vi "ViGmentize.vi"() -> ()   [LabVIEW 2025]
panel:
  in  "Style":T1(ring)=enum."material"
  in  "ACTION":bool
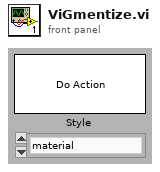
[diagram p1: front panel]
types:
  T1 = enum16{"abap", "algol", "algol_nu", "arduino", "autumn", "bw", "borland", "coffee", "colorful", "default", "dracula", "emacs", "friendly_grayscale", "friendly", "fruity", "github-dark", "gruvbox-dark", "gruvbox-light", "igor", "inkpot", "lightbulb", "lilypond", "lovelace", "manni", "material", "monokai", "murphy", "native", "nord-darker", "nord", "one-dark", "paraiso-dark", "paraiso-light", "pastie", "perldoc", "rainbow_dash", "rrt", "sas", "solarized-dark", "solarized-light", "staroffice", "stata-dark", "stata-light", "tango", "trac", "vim", "vs", "xcode", "zenburn"}
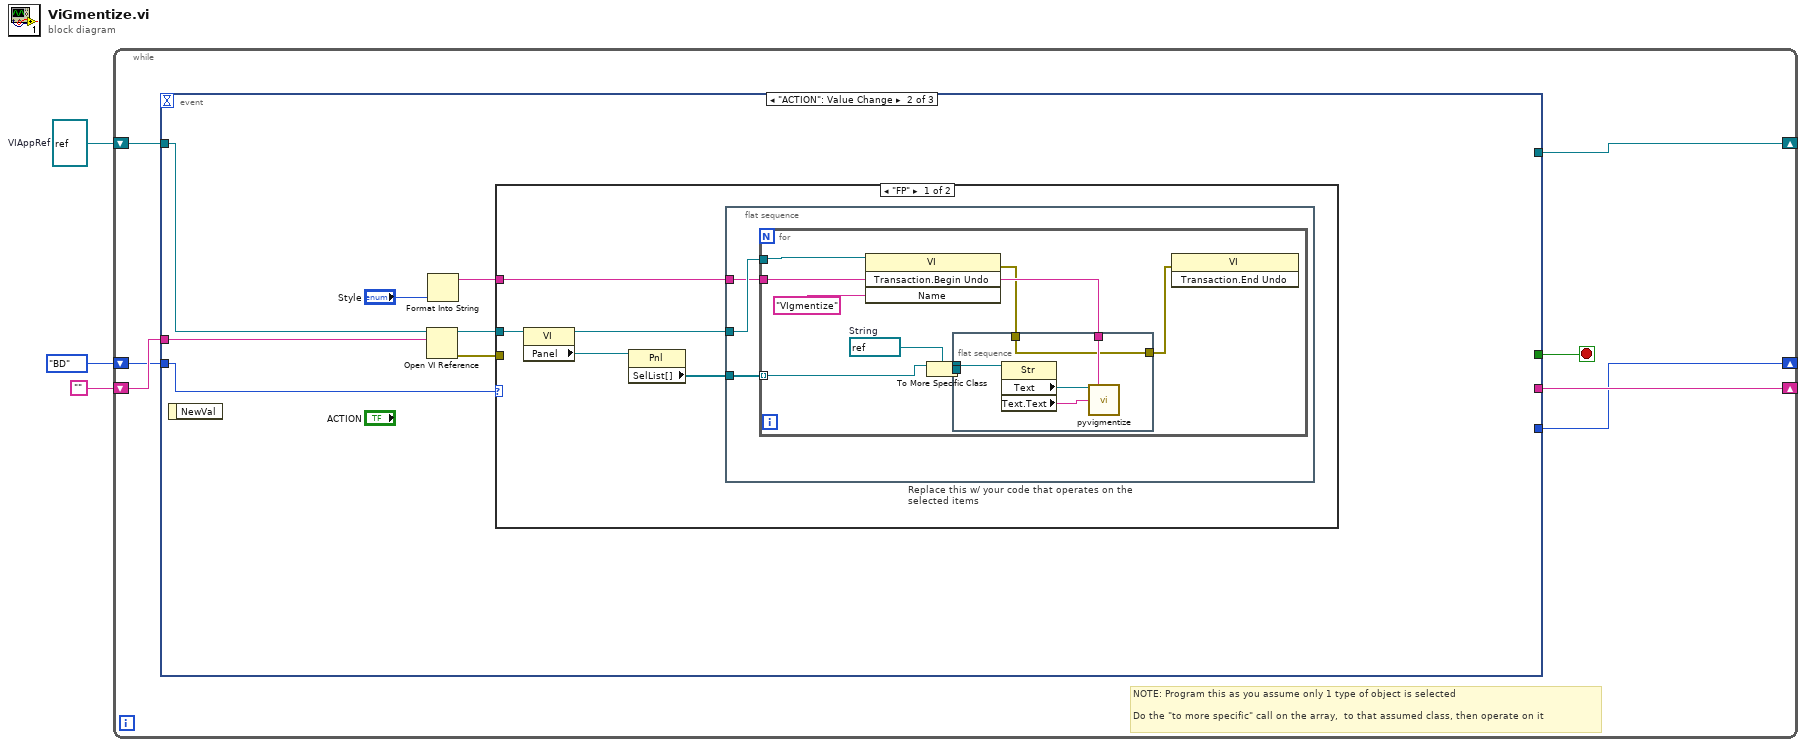
[diagram p0: block diagram]
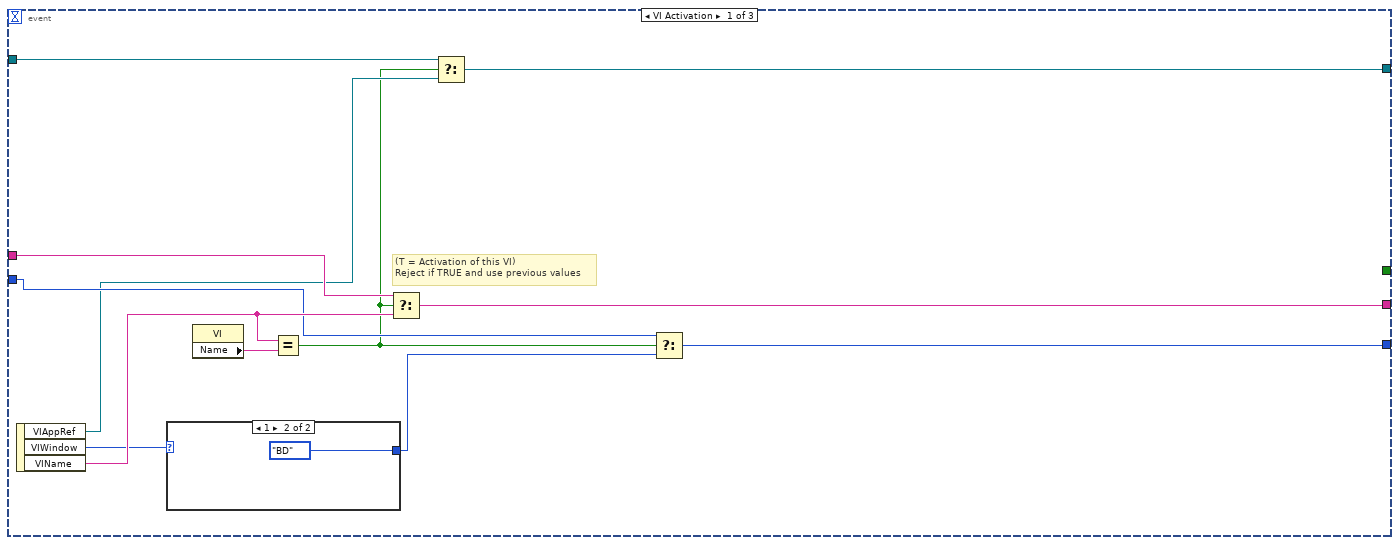
[diagram p2: hidden frame]
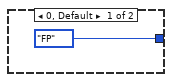
[diagram p3: hidden frame]
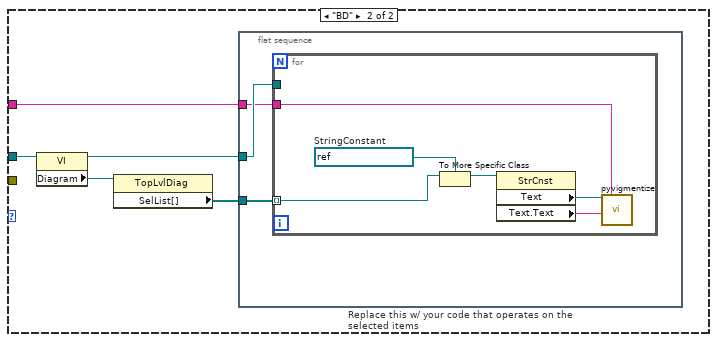
[diagram p4: hidden frame]
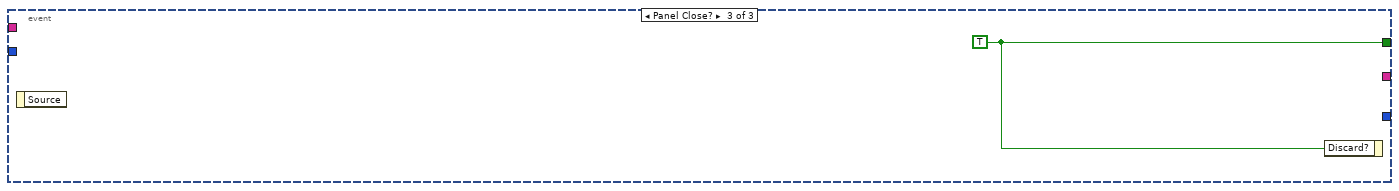
[diagram p5: hidden frame]
diagram:
  w1 = refnum<vi> refnum  # VIAppRef
  n1 = while {
    shift-right: [w10] -> _
    shift-left: "" -> [w9]
    shift-right: [w7] -> _
    shift-left: enum16{"FP", "BD"}."BD" -> [w6]
    shift-right: [w5] -> _
    shift-left: w1 -> [w4]
    stop <- w8 stop-if-true
    # "NOTE: Program this as you assume only 1 type of object is selected\n\nDo the \"to more specific\" call on the array,  to that assumed class, then operate on it"
    n2 = event shown="[1] \"ACTION\": Value Change" {
      selector: _ -> [_ _ _]
      dyn-events: _ -> [_ _ _]
      timeout: _ -> [_ _ _]
      tunnel: [w19 _ _] -> w10
      tunnel: w9 -> [w22 w31 _]
      tunnel: [_ _ w68] -> w8
      tunnel: [w17 _ _] -> w7
      tunnel: w6 -> [w18 w29 _]
      tunnel: [w13 _ _] -> w5
      tunnel: w4 -> [w12 w28 _]
      event VI Activation {
        # "(T = Activation of this VI)\nReject if TRUE and use previous values"
        n3 = event-data() -> ("VIAppRef"=w14:refnum<vi>, "VIWindow"=w16:i32, "VIName"=w20:string)  [unwired: 1 out]
        n4 = case shown="1" w16 {
          tunnel: [enum16{"FP", "BD"}."FP" enum16{"FP", "BD"}."BD"] -> w15
          frame 0, Default {
          }
          frame 1 {
          }
        }
        n5 = property class="VI"() -> ("Name"=w21:string)  [unwired: 2 in, 2 out]
        n6 = Equal?(x=w20, y=w21) -> (x = y?=w11:bool)
        n7 = Select(t=w22, s=w11, f=w20) -> (s? t:f=w19:string)
        n8 = Select(t=w12, s=w11, f=w14) -> (s? t:f=w13:refnum<vi>)
        n9 = Select(t=w18, s=w11, f=w15) -> (s? t:f=w17:enum16{"FP", "BD"})
      }
      event "ACTION": Value Change {
        n10 = event-data() -> ()  [unwired: 2 out]
        n11 = Open VI Reference(application reference (local)=w28, vi path=w31) -> (vi reference=w30:refnum<vi>, error out=w25:errorcluster)  [unwired: 2 in, 2 out]
        n12 = Format Into String("Style") -> (resulting string=w26:string)  [unwired: 3 in, 1 out]
        n13 = case shown="\"FP\"" w29 {
          tunnel: w30 -> [w36 w58]
          tunnel: w26 -> [w32 w54]
          tunnel: w25 -> [_ _]
          frame "FP" {
            n14 = property class="VI"(reference=w36) -> (reference out=w33:refnum<vi>, "Panel"=w35:refnum<vi>)  [unwired: 1 in, 1 out]
            n15 = property class="Pnl"(reference=w35) -> ("SelList[]"=w34:refnum<vi>[])  [unwired: 1 in, 2 out]
            n16 = flat-sequence "Replace this w/ your code that operates on the selected items" {
              tunnel: w34 -> [w39]
              tunnel: w33 -> [w38]
              tunnel: w32 -> [w37]
              frame #0 {
                n17 = for {
                  tunnel: w39 -> [w46] mode=indexing
                  tunnel: w38 -> [w43]
                  tunnel: w37 -> [w44]
                  w45 = refnum<vi> refnum  # String
                  n18 = invoke class="VI" method="Transaction.Begin Undo"(reference=w43, "Name"="VIgmentize") -> (error out=w41:errorcluster)  [unwired: 2 in, 3 out]
                  n19 = flat-sequence {
                    tunnel: w46 -> [w53]
                    tunnel: w45 -> [w52]
                    tunnel: w44 -> [w48]
                    tunnel: w41 -> [w47]
                    tunnel: [w47] -> w40
                    frame #0 {
                      n20 = To More Specific Class(target class=w52, reference=w53) -> (specific class reference=w51:refnum<vi>)  [unwired: 1 in, 1 out]
                      n21 = property class="Str"(reference=w51) -> ("Text"=w50:refnum<vi>, "Text.Text"=w49:string)  [unwired: 1 in, 2 out]
                      n22 = call "pyvigmentize.vi"("Text Field Destination"=w50, "style name (material)"=w48, "String"=w49) -> ()  [unwired: 13 in]
                    }
                  }
                  n23 = invoke class="VI" method="Transaction.End Undo"(error in=w40) -> ()  [unwired: 2 in, 3 out]
                }
              }
            }
          }
          frame "BD" {
            n24 = property class="VI"(reference=w58) -> (reference out=w55:refnum<vi>, "Diagram"=w57:refnum<vi>)  [unwired: 1 in, 1 out]
            n25 = property class="TopLvlDiag"(reference=w57) -> ("SelList[]"=w56:refnum<vi>[])  [unwired: 1 in, 2 out]
            n26 = flat-sequence "Replace this w/ your code that operates on the selected items" {
              tunnel: w56 -> [w61]
              tunnel: w55 -> [w60]
              tunnel: w54 -> [w59]
              frame #0 {
                n27 = for {
                  tunnel: w61 -> [w67] mode=indexing
                  tunnel: w60 -> [_]
                  tunnel: w59 -> [w62]
                  w66 = refnum<vi> refnum  # StringConstant
                  n28 = To More Specific Class(target class=w66, reference=w67) -> (specific class reference=w65:refnum<vi>)  [unwired: 1 in, 1 out]
                  n29 = property class="StrCnst"(reference=w65) -> ("Text"=w64:refnum<vi>, "Text.Text"=w63:string)  [unwired: 1 in, 2 out]
                  n30 = call "pyvigmentize.vi"("Text Field Destination"=w64, "style name (material)"=w62, "String"=w63) -> ()  [unwired: 13 in]
                }
              }
            }
          }
        }
      }
      event Panel Close? {
        w68 = TRUE ("Discard?")
        n31 = event-data() -> ()  [unwired: 2 out]
        n32 = event-data("Discard?"=w68) -> ()  [unwired: 1 in, 1 out]
      }
    }
  }
